vi "Write color.vi"(8 "error in (no error)":errorcluster, 10 "color":T1, 11 "Shape in":refnum<class "Shape.lvclass">) -> (0 "error out":errorcluster, 3 "Shape out":refnum<class "Shape.lvclass">)   [LabVIEW 2015, in "Shape.lvclass"]
uses:
  Shape.lvclass
  colors.ctl
  Shape.lvclass/Shape.ctl
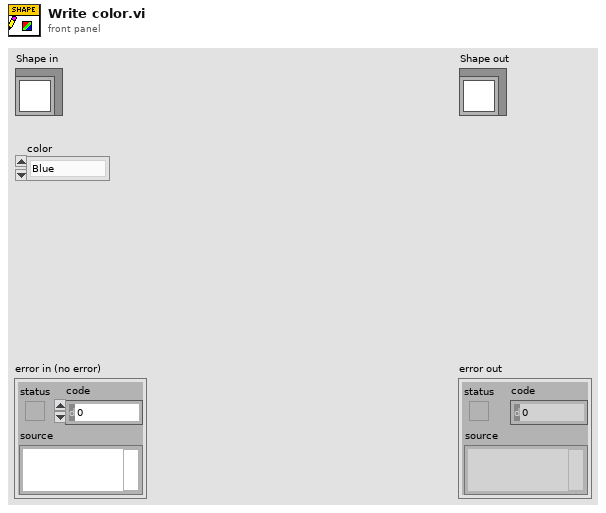
[diagram p1: front panel]
types:
  T1 = typedef "colors.ctl" = enum16{"Blue", "Red", "Green", "Yellow"}
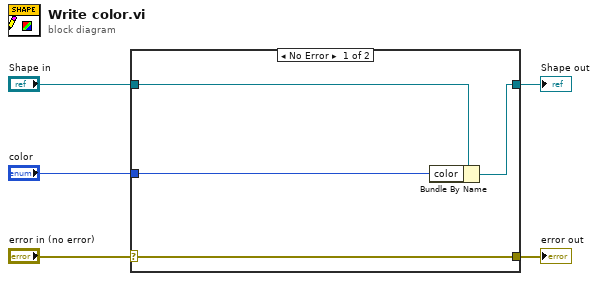
[diagram p0: block diagram]
diagram:
  n1 = case shown="No Error" "error in (no error)" {
    selector: "error in (no error)" -> [w9 w10]
    tunnel: [w9 w10] -> w4
    tunnel: [w7 w11] -> w2
    tunnel: "Shape in" -> [w8 w11]
    tunnel: "color" -> [w6 _]
    frame No Error {
      n2 = Bundle By Name(cluster=w8, "color"=w6) -> (w7:refnum<class "Shape.lvclass">)
    }
    frame Error {
    }
  }
  "error out" <- w4
  "Shape out" <- w2
